vi "susp_subvi.vi"(11 "Numeric in":fxp<+,32,3>) -> (3 "Numeric out":sgl)   [LabVIEW 2014]
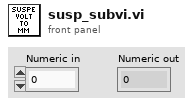
[diagram p1: front panel]
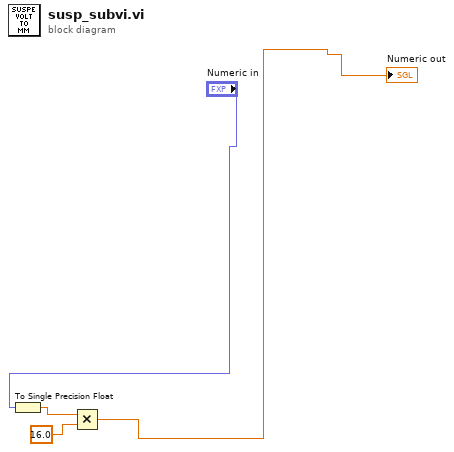
[diagram p0: block diagram]
diagram:
  n1 = To Single Precision Float(number="Numeric in") -> (single precision float=w3:sgl)
  n2 = Multiply(x=w3, y=sgl 16.0) -> (x*y=→"Numeric out":sgl)
